vi "Freq Peak.vi"(8 "error in (no error)":errorcluster, 11 "Instrument Handle In":refnum<k21>) -> (0 "error out":errorcluster, 1 "Peak Frequency (Hz)":dbl format="%.6p", 2 "Peak Amplitude":dbl format="%.2f", 3 "Instrument Handle Out":refnum<k21>)   [LabVIEW 2018]
uses:
  <vilib>/RFmx/SpecAn/mx/RFmxSpecAn.llb/RFmxSpecAn Spectrum Fetch Measurement.vi
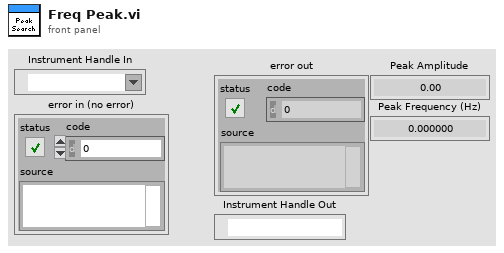
[diagram p1: front panel]
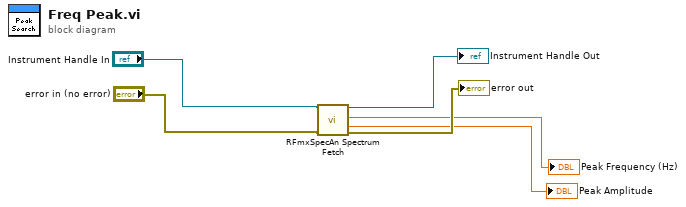
[diagram p0: block diagram]
diagram:
  n1 = call-poly <vilib>:"RFmxSpecAn Spectrum Fetch.vi"("Instrument Handle In"="Instrument Handle In", "error in (no error)"="error in (no error)") -> ("Instrument Handle Out"=→"Instrument Handle Out":refnum<k21>, "Peak Amplitude"=→"Peak Amplitude":dbl, "Peak Frequency (Hz)"=→"Peak Frequency (Hz)":dbl, "error out"=→"error out":errorcluster)  [unwired: 9 in, 1 out]
